vi "Build Data Frame.vi"(0 "RFFE RegWriteExt Command in":refnum<class "RFFE RegWriteExt Command.lvclass">, 11 "error in (no error)":errorcluster) -> (4 "RFFE RegWriteExt Command out":refnum<class "RFFE RegWriteExt Command.lvclass">, 6 "Data Frame":u8[](array[numeric]), 15 "error out":errorcluster)   [LabVIEW 2018, in "MIPI RFFE API.lvlib" / "RFFE RegWriteExt Command.lvclass"]
uses:
  RFFE RegWriteExt Command.lvclass
  C:/Users/semoore/Projects/mipi-rffe-labview-oop/Extended Command/RFFE Extended Command.lvclass
  Extended Command/RFFE Extended Command.lvclass/RFFE Extended Command.ctl
  Extended Command/Get Register Data.vi
  MIPI RFFE API.lvlib
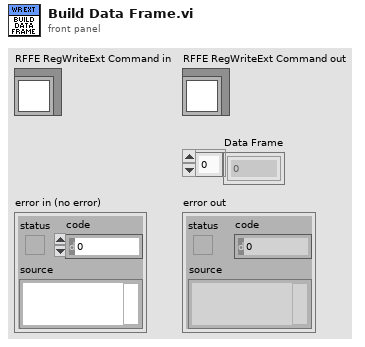
[diagram p1: front panel]
types:
  T1 = typedef "RFFE Commands.lvlib/Register Data.ctl" = u8
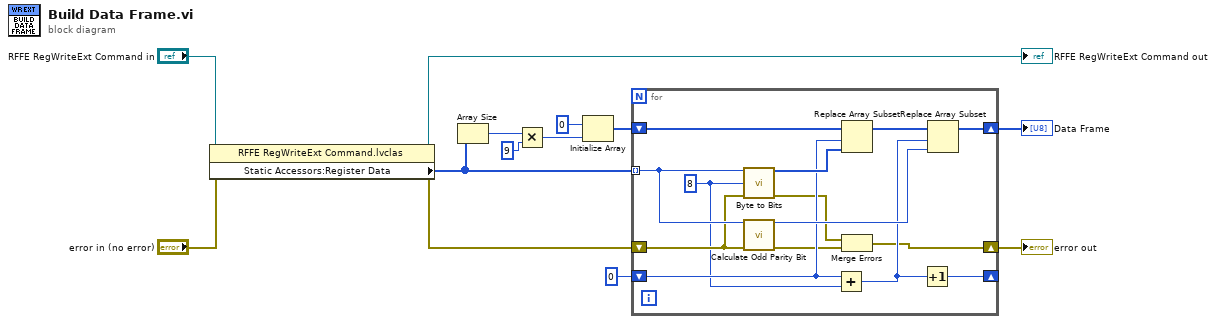
[diagram p0: block diagram]
diagram:
  n1 = property class="RFFE RegWriteExt Command.lvclas"(reference="RFFE RegWriteExt Command in", error in="error in (no error)") -> (reference out=→"RFFE RegWriteExt Command out":refnum<class "RFFE RegWriteExt Command.lvclass">, error out=w1:errorcluster, "Static Accessors:Register Data"=w2:T1[])
  n2 = Array Size(array=w2) -> (size(s)=w7:i32)
  n3 = Multiply(x=w7, y=9) -> (x*y=w5:i32)
  n4 = Initialize Array(u8 0 ("Register Data"), w5) -> (w4:u8[])
  n5 = for {
    tunnel: w2 -> [w27] mode=indexing
    shift-right: [w14] -> w12
    shift-left: w1 -> [w26]
    shift-right: [w25] -> w13
    shift-left: w4 -> [w22]
    shift-right: [w18] -> _
    shift-left: 0 -> [w20]
    w17 = 8 ("Bit Width")
    n6 = call "Byte to Bits.vi"("Byte"=w27, "Bit Width"=w17, "error in (no error)"=w26) -> ("Bits"=w23:u8[], "error out"=w15:errorcluster)  [unwired: 11 in]
    n7 = call "Calculate Odd Parity Bit.vi"("Byte"=w27, "error in (no error)"=w26) -> ("Odd Parity Bit"=w24:u8, "error out"=w16:errorcluster)  [unwired: 12 in]
    n8 = Add(x=w20, y=w17) -> (x+y=w19:i32)
    n9 = Replace Array Subset(array=w22, new element=w23, index=w20) -> (w21:u8[])
    n10 = Merge Errors(w15, w16) -> (w14:errorcluster)
    n11 = Increment(x=w19) -> (x+1=w18:i32)
    n12 = Replace Array Subset(array=w21, new element=w24, index=w19) -> (w25:u8[])
  }
  "error out" <- w12
  "Data Frame" <- w13
